vi "FTW-STR-Random-Bytes.vi"(3 "String Length":i32=32) -> (0 "Random Bytes":string)   [LabVIEW 2015]
panel:
  # "Inputs"
  # "Outputs"
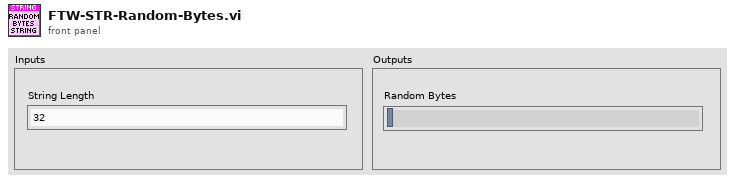
[diagram p1: front panel]
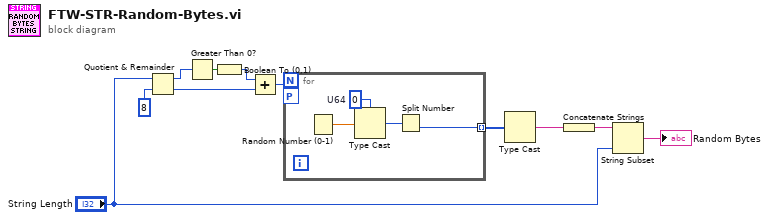
[diagram p0: block diagram]
diagram:
  n1 = Quotient & Remainder(x="String Length", y=8) -> (x-y*floor(x/y)=w7:i32, floor(x/y)=w4:i32)
  n2 = Greater Than 0?(x=w7) -> (x > 0?=w6:bool)
  n3 = Boolean To (0,1)(Boolean=w6) -> (0, 1=w5:i16)
  n4 = Add(x=w5, y=w4) -> (x+y=w3:i32)
  n5 = for {
    N: w3 -> [_]
    tunnel: [w12] -> w2 mode=indexing
    workers-P: _ -> [_]
    w14 = u64 0  # U64
    n6 = Random Number (0-1)() -> (number: 0 to 1=w15:dbl)
    n7 = Type Cast(type=w14, x=w15) -> (*(type *) &x=w13:u64)
    n8 = Split Number(x=w13) -> (lo(x)=w12:u32)  [unwired: 1 out]
  }
  n9 = Type Cast(x=w2) -> (*(type *) &x=w1:string)  [unwired: 1 in]
  n10 = Concatenate Strings(w1) -> (w8:string)
  n11 = String Subset(string=w8, length (rest)="String Length") -> (substring=→"Random Bytes":string)  [unwired: 1 in]
